vi "sendValue.vi"(8 "error in (no error)":errorcluster, 10 "data":variant, 11 "loopTimeOutOfRange in":refnum<class "loopTimeOutOfRange.lvclass">) -> (0 "error out":errorcluster, 2 "function return":i32, 3 "loopTimeOutOfRange out":refnum<class "loopTimeOutOfRange.lvclass">)   [LabVIEW 2016, in "SALLV_EXA_Messaging.lvlib" / "loopTimeOutOfRange.lvclass"]
uses:
  loopTimeOutOfRange.lvclass
  ts_sallv_MtAtElectrometer/DataTypes/logevent_loopTimeOutOfRange.ctl
  loopTimeOutOfRange.lvclass/loopTimeOutOfRange.ctl
  ts_sallv_MtAtElectrometer/SALLV_MtAtElectrometer.lvlib
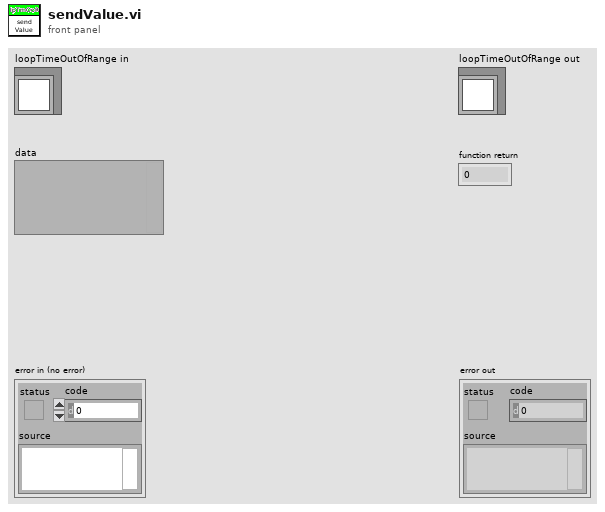
[diagram p1: front panel]
types:
  T1 = typedef "SALLV_MtAtElectrometer.lvlib/logevent_loopTimeOutOfRange.ctl" = cluster{"loopTimeOutOfRange":bool, "priority":i32}
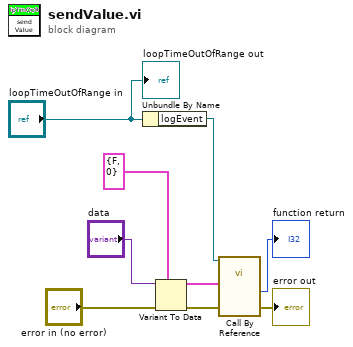
[diagram p0: block diagram]
diagram:
  n1 = Unbundle By Name("loopTimeOutOfRange in") -> ("logEvent"=w7:refnum<vi>)
  n2 = Variant To Data(error in="error in (no error)", type=T1 {"loopTimeOutOfRange"=FALSE, "priority"=0} ("logevent_loopTimeOutOfRange"), Variant="data") -> (data=w1:T1, error out=w5:errorcluster)
  n3 = call-by-ref "?"(reference=w7, "error in (no error)"=w5, "logevent_heartbeat_Ctl"=w1) -> ("error out"=→"error out":errorcluster, "function return"=→"function return":i32)  [unwired: 8 in, 3 out]
  "loopTimeOutOfRange out" <- "loopTimeOutOfRange in"
